vi "Initialize Array.vi"() -> ()   [LabVIEW 2017]
panel:
  out "initialized array 2":dbl[][][][](array[numeric])
  in  "dimension size":i32
  in  "element":dbl
  # "Review this one"
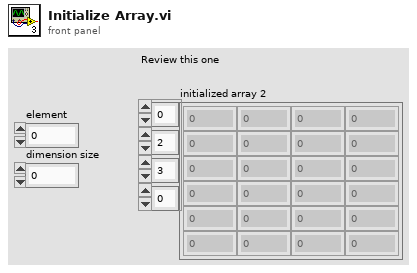
[diagram p1: front panel]
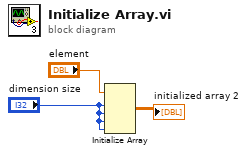
[diagram p0: block diagram]
diagram:
  n1 = Initialize Array("element", "dimension size", "dimension size", "dimension size", "dimension size") -> (→"initialized array 2":dbl[][][][])
